vi "writeFile RawTestData.vi"(6 "Test Results":T1, 8 "Session Info":T2={"V set"=-1.0, "I compliance"=0.001, "J set"=0.01, "I set"=0.0, "V compliance"=1.0, "Laser Power (mW)"=0.0, "TestID"=0, "Session Time"=timestamp(0 s since 1904-01-01), "Operator"="Radek"} {"V compliance" format="%#_6f"; "I compliance" format="%#_6e"}, 9 "Die Info":T3={"Device Name"="", "ActiveArea_um2"=3848.451, "MesaArea_um2"=3848.451, "x"=0.0, "y"=0.0}, 10 "Wafer Info":T4, 11 "Path":path) -> (3 "Path out":path)   [LabVIEW 2012]
uses:
  <vilib>/Utility/file.llb/Write To Spreadsheet File (string).vi
panel:
  out "Data Array":string[](array[string])
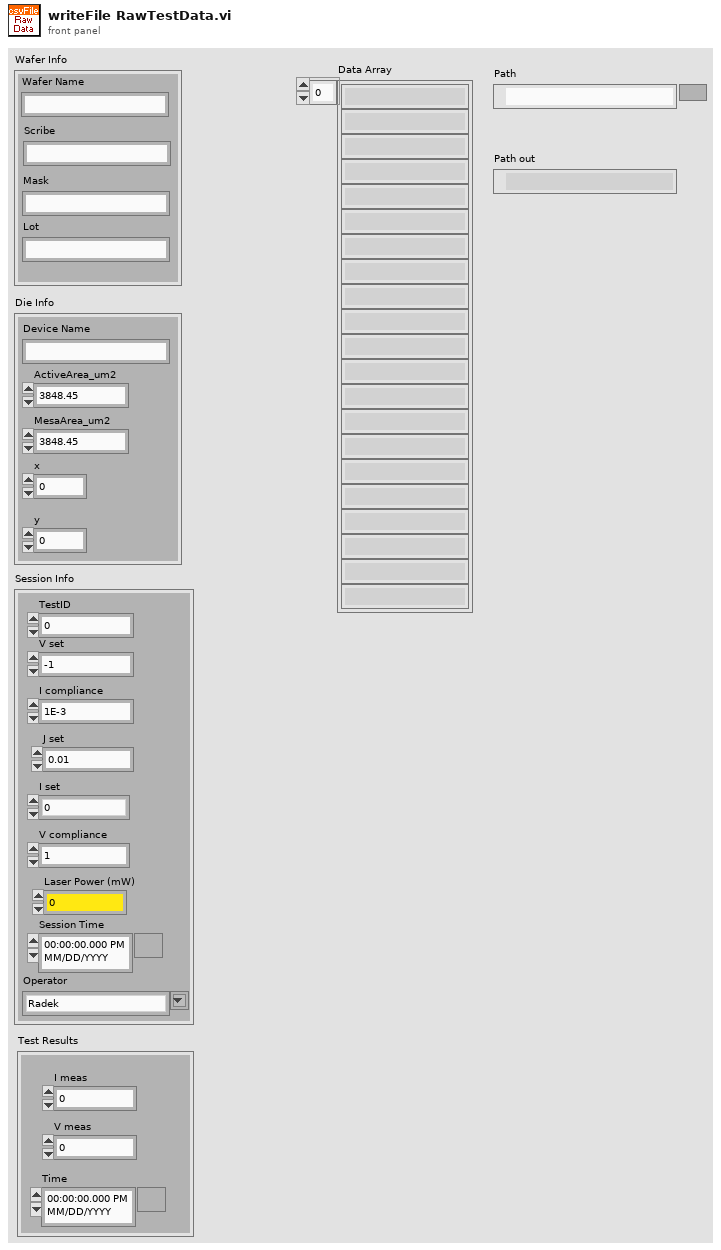
[diagram p1: front panel]
types:
  T1 = cluster{"I meas":dbl, "V meas":dbl, "Time":timestamp}
  T2 = cluster{"V set":dbl, "I compliance":dbl, "J set":dbl, "I set":dbl, "V compliance":dbl, "Laser Power (mW)":dbl, "TestID":u32, "Session Time":timestamp, "Operator":string}
  T3 = cluster{"Device Name":string, "ActiveArea_um2":dbl, "MesaArea_um2":dbl, "x":dbl, "y":dbl}
  T4 = cluster{"Wafer Name":string, "Scribe":string, "Mask":string, "Lot":string}
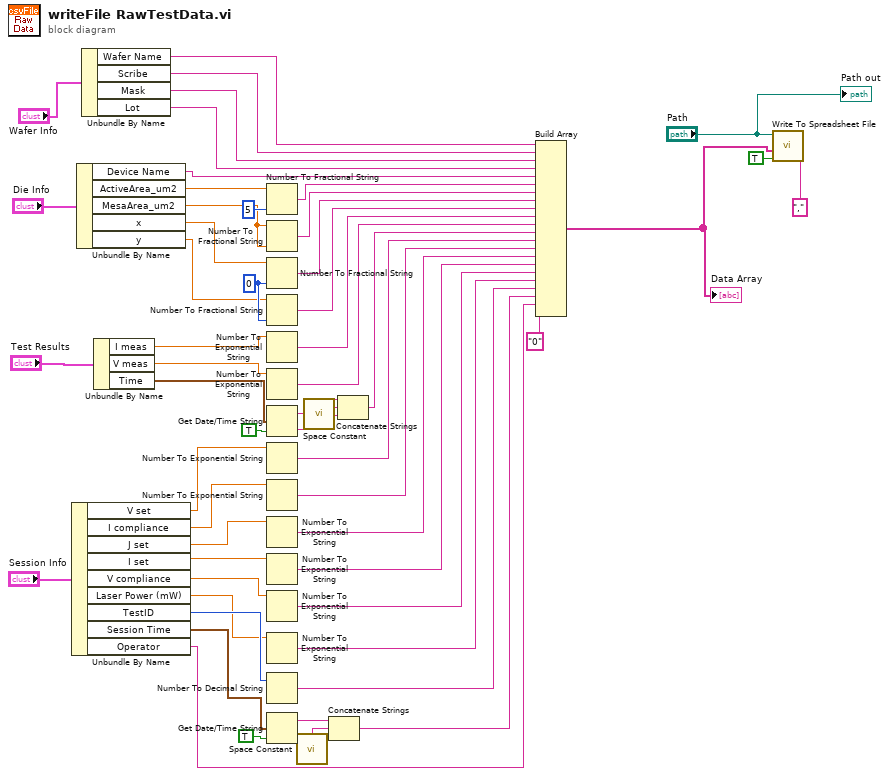
[diagram p0: block diagram]
diagram:
  w42 = i16 0 ("precision (6)")
  n1 = Unbundle By Name("Session Info") -> ("V set"=w33:dbl, "I compliance"=w24:dbl, "J set"=w23:dbl, "I set"=w22:dbl, "V compliance"=w21:dbl, "Laser Power (mW)"=w7:dbl, "TestID"=w20:u32, "Session Time"=w14:timestamp, "Operator"=w10:string)
  n2 = Unbundle By Name("Die Info") -> ("Device Name"=w47:string, "ActiveArea_um2"=w46:dbl, "MesaArea_um2"=w44:dbl, "x"=w43:dbl, "y"=w41:dbl)
  n3 = Unbundle By Name("Wafer Info") -> ("Wafer Name"=w54:string, "Scribe"=w53:string, "Mask"=w52:string, "Lot"=w51:string)
  n4 = Unbundle By Name("Test Results") -> ("I meas"=w40:dbl, "V meas"=w39:dbl, "Time"=w38:timestamp)
  n5 = Number To Fractional String(number=w46, precision (6)=i16 5) -> (F-format string=w32:string)  [unwired: 2 in]
  n6 = Number To Fractional String(number=w44, precision (6)=w44) -> (F-format string=w31:string)  [unwired: 2 in]
  n7 = Number To Fractional String(number=w43, precision (6)=w42) -> (F-format string=w30:string)  [unwired: 2 in]
  n8 = Number To Fractional String(number=w41, precision (6)=w42) -> (F-format string=w29:string)  [unwired: 2 in]
  n9 = Number To Exponential String(number=w40) -> (E-format string=w28:string)  [unwired: 3 in]
  n10 = Number To Exponential String(number=w39) -> (E-format string=w27:string)  [unwired: 3 in]
  n11 = Get Date/Time String(seconds (now)=w38, want seconds? (F)=TRUE) -> (date string=w36:string, time string=w34:string)  [unwired: 1 in]
  n12 = Number To Exponential String(number=w33) -> (E-format string=w25:string)  [unwired: 3 in]
  n13 = Number To Exponential String(number=w24) -> (E-format string=w19:string)  [unwired: 3 in]
  n14 = Number To Exponential String(number=w23) -> (E-format string=w18:string)  [unwired: 3 in]
  n15 = Number To Exponential String(number=w22) -> (E-format string=w17:string)  [unwired: 3 in]
  n16 = Number To Exponential String(number=w21) -> (E-format string=w16:string)  [unwired: 3 in]
  n17 = Number To Exponential String(number=w7) -> (E-format string=w6:string)  [unwired: 3 in]
  n18 = Number To Decimal String(number=w20) -> (decimal integer string=w8:string)  [unwired: 1 in]
  n19 = Get Date/Time String(seconds (now)=w14, want seconds? (F)=TRUE) -> (date string=w13:string, time string=w12:string)  [unwired: 1 in]
  n20 = call <vilib>:"Space Constant.vi"() -> ("String"=w11:string)
  n21 = call <vilib>:"Space Constant.vi"() -> ("String"=w35:string)
  n22 = Concatenate Strings(w13, w11, w12) -> (w9:string)
  n23 = Concatenate Strings(w36, w35, w34) -> (w26:string)
  n24 = Build Array(w54, w53, w52, w51, w47, w32, w31, w30, w29, w28, w27, w26, w25, w19, w18, w17, w16, w6, w8, w9, w10, "0" ("element")) -> (w5:string[])
  "Data Array" <- w5
  n25 = call-poly <vilib>:"Write To Spreadsheet File.vi"("delimiter (\\t)"="," ("delimiter (\\t)"), "append to file? (new file:F)"=TRUE, "1D data"=w5, "file path (dialog if empty)"="Path") -> ()  [unwired: 4 in, 1 out]
  "Path out" <- "Path"
